vi "Add Calculate Channel_Acceleration_Acceleration.vi"(7 "SysDef Ref":T1, 8 "error in (error out)":errorcluster, 9 "Acceleration Settings":T2, 11 "Calculated Channels Ref":refnum<k24>) -> (0 "error out":errorcluster, 3 "Calculated Channels Ref Out":refnum<k24>)   [LabVIEW 2019, in "Simple SysDef API.lvlib"]
uses:
  <userlib>/SimpleSysDef/Simple SysDef API.lvlib
  NationalInstruments.VeriStand.SystemDefinitionAPI
  <userlib>/SimpleSysDef/_SubVIs/Add Calculate Channel_Acceleration_Settings.ctl
  <userlib>/SimpleSysDef/_SubVIs/System Definition Reference.ctl
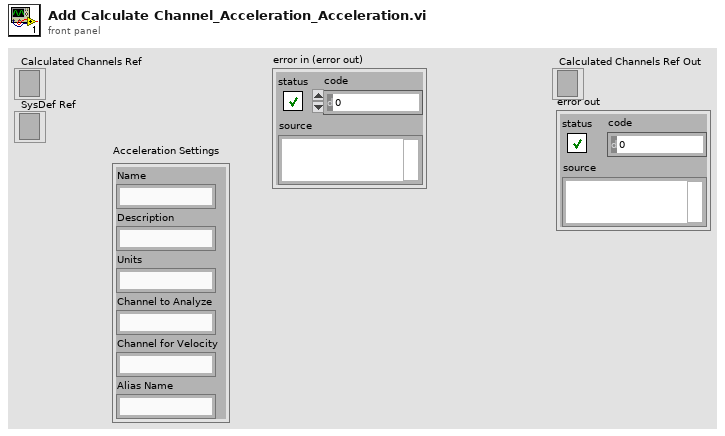
[diagram p1: front panel]
types:
  T1 = typedef "Simple SysDef API.lvlib/System Definition Reference.ctl" = refnum<k24>
  T2 = typedef "Simple SysDef API.lvlib/Add Calculate Channel_Acceleration_Settings.ctl" = cluster{"Name":string, "Description":string, "Units":string, "Channel to Analyze":string, "Channel for Velocity":string, "Alias Name":string}
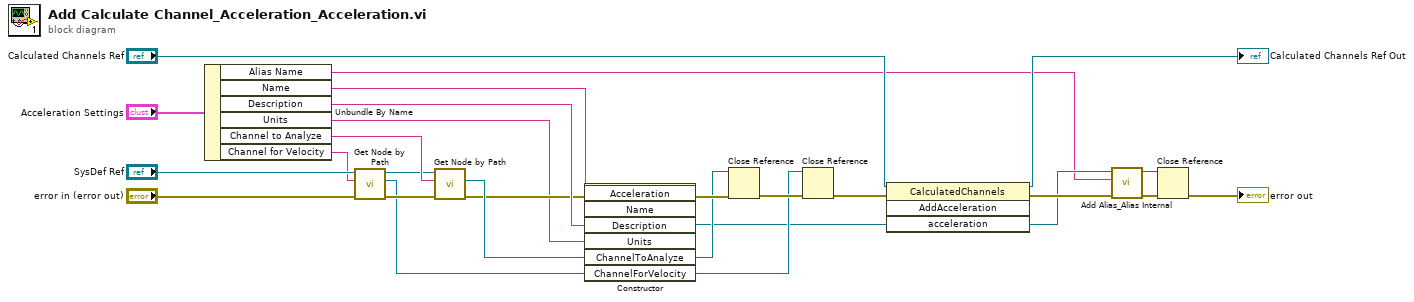
[diagram p0: block diagram]
diagram:
  n1 = Unbundle By Name("Acceleration Settings") -> ("Alias Name"=w1:string, "Name"=w19:string, "Description"=w18:string, "Units"=w10:string, "Channel to Analyze"=w17:string, "Channel for Velocity"=w9:string)
  n2 = call <userlib>:"Get Node by Path.vi"("error in (no error)"="error in (error out)", "System Definition Node Path"=w9, "SysDef Ref"="SysDef Ref") -> ("error out"=w13:errorcluster, "Node Ref"=w6:refnum<k24>, "SysDef Ref Out"=w11:T1)  [unwired: 6 in]
  n3 = call <userlib>:"Get Node by Path.vi"("error in (no error)"=w13, "System Definition Node Path"=w17, "SysDef Ref"=w11) -> ("error out"=w15:errorcluster, "Node Ref"=w16:refnum<k24>)  [unwired: 6 in, 1 out]
  n4 = constructor class="Acceleration"(error in=w15, "Name"=w19, "Description"=w18, "Units"=w10, "ChannelToAnalyze"=w16, "ChannelForVelocity"=w6) -> (reference out=w2:refnum<k24>, error out=w20:errorcluster)  [unwired: 2 in, 6 out]
  n5 = Close Reference(reference=w16, error in (no error)=w20) -> (error out=w8:errorcluster)
  n6 = Close Reference(reference=w6, error in (no error)=w8) -> (error out=w7:errorcluster)
  n7 = invoke class="CalculatedChannels" method="AddAcceleration"(reference="Calculated Channels Ref", error in=w7, "acceleration"=w2) -> (reference out=→"Calculated Channels Ref Out":refnum<k24>, error out=w5:errorcluster)  [unwired: 1 in, 2 out]
  n8 = call <userlib>:"Add Alias_Alias Internal.vi"("error in (no error)"=w5, "Name"=w1, "Base Node"=w2) -> ("error out"=w4:errorcluster, "Base Node out"=w3:refnum<k24>)  [unwired: 7 in]
  n9 = Close Reference(reference=w3, error in (no error)=w4) -> (error out=→"error out":errorcluster)
